vi "Initialization VI.vi"(8 "error in (no error)":errorcluster, 10 "Custom XML":string, 11 "Device Item Ref in":T1 format="%.0x") -> (0 "error out":errorcluster, 3 "Device Ref out":T1 format="%.0x")   [LabVIEW 2013, in "PWM System Explorer.lvlib"]
uses:
  PWM System Explorer.lvlib
  <vilib>/NI Veristand/Custom Device API/Custom Device Item Ref.ctl
  <vilib>/NI Veristand/Custom Device API/Custom Device Loop Type.ctl
  Shared/Constants.vi
  <vilib>/NI Veristand/Custom Device API/Set Item Property (String).vi
  <vilib>/NI Veristand/Custom Device API/Set Item Property (Variant).vi
  <vilib>/NI Veristand/Custom Device API/Custom Device API.lvlib
  Shared/PWM Shared.lvlib
  <vilib>/NI Veristand/Custom Device Tools/Custom Device Utility Library/Custom Device Utility Library.lvlib
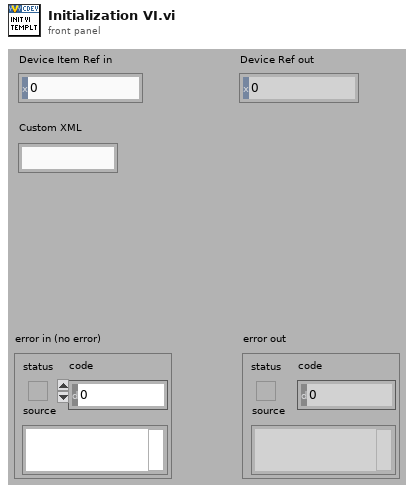
[diagram p1: front panel]
types:
  T1 = typedef "Custom Device API.lvlib/Custom Device Item Ref.ctl" = u64
  T2 = typedef "Custom Device API.lvlib/Custom Device Loop Type.ctl" = enum32{"While Loop", "Timed Loop"}
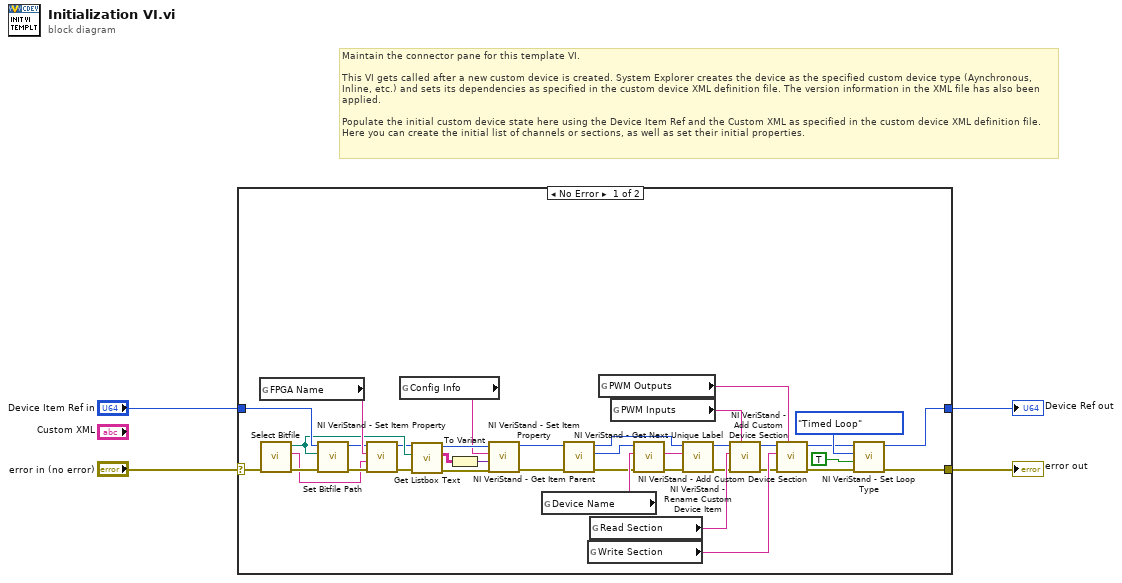
[diagram p0: block diagram]
diagram:
  # "Maintain the connector pane for this template VI.\n\nThis VI gets called after a new custom device is created. System Explorer creates the device as the specified custom device type (Aynchronous, Inline, etc.) and sets its dependencies as specified in the custom device XML definition file. The version information in the XML file has also been applied.\n\nPopulate the initial custom device state here using the Device Item Ref and the Custom XML as specified in the custom device XML definition file. Here you can create the initial list of channels or sections, as well as set their initial properties."
  n1 = case shown="No Error" "error in (no error)" {
    selector: "error in (no error)" -> [w41 w42]
    tunnel: [w17 w43] -> w3
    tunnel: "Device Item Ref in" -> [w39 w43]
    tunnel: [w16 w42] -> w1
    frame No Error {
      n2 = global read "Constants.vi" "FPGA Name"() -> (w40:string)
      n3 = call "Select Bitfile.vi"("error in"=w41) -> ("error out"=w38:errorcluster, "RIO Device Address out"=w21:string, "Bitfile Path out"=w13:path)  [unwired: 7 in, 1 out]
      n4 = call "Set Bitfile Path.vi"("error in (no error)"=w38, "Bitfile Path in"=w13, "Device Ref in"=w39) -> ("error out"=w22:errorcluster, "Device Ref out"=w23:T1)  [unwired: 7 in]
      n5 = call-poly <vilib>:"NI VeriStand - Set Item Property.vi"("error in (no error)"=w22, "Value"=w21, "Property Name"=w40, "Item Ref in"=w23) -> ("error out"=w8:errorcluster, "Item Ref out"=w10:T1)  [unwired: 5 in, 1 out]
      n6 = global read "Constants.vi" "Config Info"() -> (w7:string)
      n7 = call "Get Listbox Text.vi"("error in (no error)"=w8, "bitfile path"=w13, "Node Ptr"=w10) -> ("error out"=w14:errorcluster, "Control Info"=w6:string[][], "Node Ptr out"=w12:T1)  [unwired: 6 in]
      n8 = To Variant(anything=w6) -> (Variant=w5:variant)
      n9 = call-poly <vilib>:"NI VeriStand - Set Item Property.vi"("error in (no error)"=w14, "Value"=w5, "Property Name"=w7, "Item Ref in"=w12) -> ("error out"=w11:errorcluster, "Item Ref out"=w9:T1)  [unwired: 5 in, 1 out]
      n10 = global read "Constants.vi" "Device Name"() -> (w37:string)
      n11 = call <vilib>:"NI VeriStand - Get Item Parent.vi"("error in (no error)"=w11, "Item Ref in"=w9) -> ("error out"=w36:errorcluster, "Parent Ref"=w35:T1, "Item Ref out"=w32:T1)  [unwired: 6 in, 1 out]
      n12 = global read "Constants.vi" "Write Section"() -> (w27:string)
      n13 = global read "Constants.vi" "Read Section"() -> (w30:string)
      n14 = global read "Constants.vi" "PWM Outputs"() -> (w28:string)
      n15 = global read "Constants.vi" "PWM Inputs"() -> (w29:string)
      n16 = call <vilib>:"NI VeriStand - Get Next Unique Label.vi"("error in (no error)"=w36, "Label"=w37, "Parent Ref in"=w35) -> ("error out"=w34:errorcluster, "Label out"=w33:string)  [unwired: 5 in, 2 out]
      n17 = call <vilib>:"NI VeriStand - Rename Custom Device Item.vi"("error in (no error)"=w34, "New Name"=w33, "Item Ref in"=w32) -> ("error out"=w25:errorcluster, "Item Ref out"=w31:T1)  [unwired: 6 in, 1 out]
      n18 = call <vilib>:"NI VeriStand - Add Custom Device Section.vi"("GUID (Default Section)"=w29, "error in (no error)"=w25, "Section Name"=w30, "Parent Ref in"=w31) -> ("error out"=w26:errorcluster, "Parent Ref out"=w24:T1)  [unwired: 4 in, 2 out]
      n19 = call <vilib>:"NI VeriStand - Add Custom Device Section.vi"("GUID (Default Section)"=w28, "error in (no error)"=w26, "Section Name"=w27, "Parent Ref in"=w24) -> ("error out"=w15:errorcluster, "Parent Ref out"=w18:T1)  [unwired: 4 in, 2 out]
      n20 = call <vilib>:"NI VeriStand - Set Loop Type.vi"("error in (no error)"=w15, "Use Device Clock (Timed Loops only)"=TRUE, "Loop type"=Custom_Device_Loop_Type."Timed Loop", "Device Ref in"=w18) -> ("error out"=w16:errorcluster, "Device Ref out"=w17:T1)  [unwired: 6 in]
    }
    frame Error {
    }
  }
  "error out" <- w1
  "Device Ref out" <- w3
